vi "ContSplitGeneralSettings.vi"(11 "General Settings":string[][](array[string])) -> (0 "Interval":timestamp, 1 "Total Duration":timestamp, 2 "File Prefix":string, 3 "SaveDir":path)   [LabVIEW 2018]
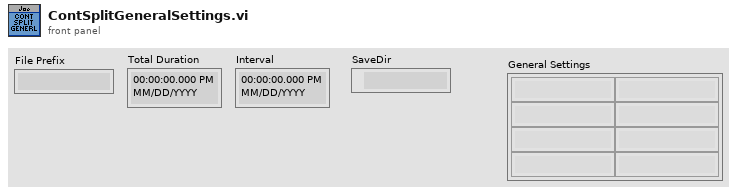
[diagram p1: front panel]
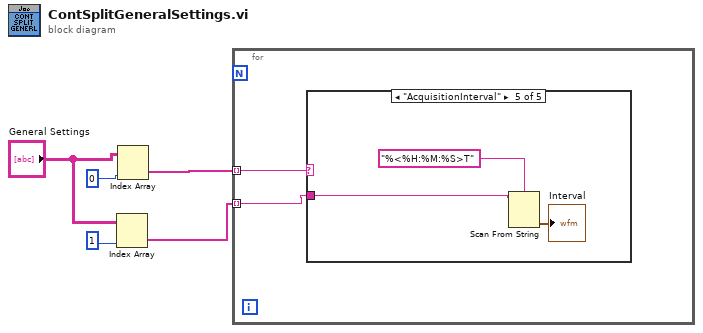
[diagram p0: block diagram]
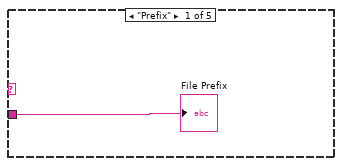
[diagram p2: hidden frame]
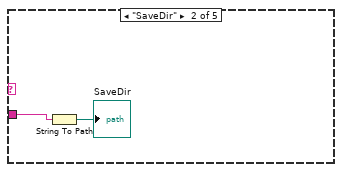
[diagram p3: hidden frame]
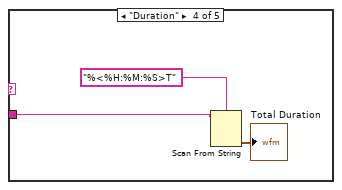
[diagram p5: hidden frame]
diagram:
  n1 = Index Array(array="General Settings", index (col)=1 ("disabled index (col)")) -> (element=w3:string[])  [unwired: 1 in]
  n2 = Index Array(array="General Settings", index (col)=0 ("index")) -> (element=w5:string[])  [unwired: 1 in]
  n3 = for {
    tunnel: w5 -> [w7] mode=indexing
    tunnel: w3 -> [w6] mode=indexing
    n4 = case shown="\"AcquisitionInterval\"" w7 {
      tunnel: w6 -> [w8 w10 _ w13 w16]
      frame "Prefix" {
        "File Prefix" <- w8
      }
      frame "SaveDir" {
        n5 = String To Path(string=w10) -> (path=→"SaveDir":path)
      }
      frame Default {
      }
      frame "Duration" {
        n6 = Scan From String(format string="%<%H:%M:%S>T", input string=w13) -> (output 1=→"Total Duration":timestamp)  [unwired: 3 in, 3 out]
      }
      frame "AcquisitionInterval" {
        n7 = Scan From String(format string="%<%H:%M:%S>T", input string=w16) -> (output 1=→"Interval":timestamp)  [unwired: 3 in, 3 out]
      }
    }
  }
